vi "RDS Child Receive Message.vi"(8 "error in (no error)":errorcluster, 10 "RDS Message":refnum<class "RDS Message.lvclass">, 11 "RDS Test Child in":refnum<class "RDS Test Child.lvclass">) -> (0 "error out":errorcluster, 3 "RDS Test Child out":refnum<class "RDS Test Child.lvclass">)   [LabVIEW 2015, in "RDS Test Child.lvlib" / "RDS Test Child.lvclass"]
uses:
  RDS Test Child.lvclass
  Libraries/RDS Framework/RDS Message Class/RDS Message.lvclass
  Libraries/RDS Framework/RDS Message Class/RDS Message.lvclass/RDS Message.ctl
  Libraries/RDS Child Messages/AIP Status Message/AIP Status Response.lvclass
  Libraries/RDS Child Messages/AIP Status Message/AIP Status Response.lvclass/AIP Status Response.ctl
  RDS Test Child.lvclass/RDS Test Child.ctl
  Libraries/RDS Child Messages/GPS Data Message/GPS Data Message.lvclass
  Libraries/RDS Child Messages/GPS Data Message/GPS Data Message.lvclass/GPS Data Message.ctl
  Libraries/RDS Child Messages/State Sample Message/State Sample Message.lvclass
  Libraries/RDS Child Messages/State Sample Message/State Sample Message.lvclass/State Sample Message.ctl
  Libraries/RDS Child Messages/Helm/Helm Status Message/Helm Status Message.lvclass
  Libraries/RDS Child Messages/Helm/Helm Status Message/Helm Status Message.lvclass/Helm Status Message.ctl
  Libraries/RDS Child Messages/Depth Data Message/Depth Data Message.lvclass
  Libraries/RDS Child Messages/Depth Data Message/Depth Data Message.lvclass/Depth Data Message.ctl
  Libraries/RDS Child Messages/Battery Data/Battery Message.lvclass
  Libraries/RDS Child Messages/Battery Data/Battery Message.lvclass/Battery Message.ctl
  Libraries/RDS Child Messages/MCB/MCB Status Message/MCB Status.lvclass
  Libraries/RDS Child Messages/MCB/MCB Status Message/MCB Status.lvclass/MCB Status.ctl
  Libraries/RDS Child Messages/Compass/Compass Data Message.lvclass
  <vilib>/Utility/miscctls.llb/LV3DPointTypeDef.ctl
  Libraries/RDS Child Messages/Compass/Compass Data Message.lvclass/Compass Data Message.ctl
  Libraries/RDS Serial Handler/RDS Serial Frame.lvclass
  RDS State Tracker/RDS State/RDS State.lvclass
  Libraries/3rd Party/Artificial Horizon/lv-attitudecontrol.lvlib
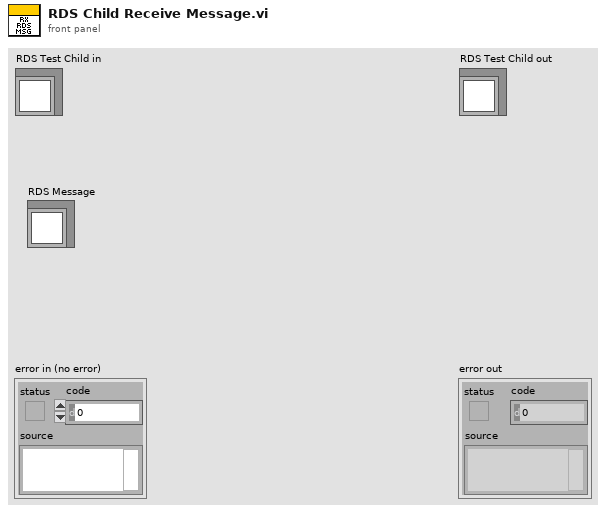
[diagram p1: front panel]
types:
  T1 = typedef "RDS Child Messages.lvlib/RDS Message ID.ctl" = enum16{"RDS Hello World", "String Message", "AIP_Status", "AIP_Command", "GPS_Data", "MCB_Command", "MCB_Status", "Compass_Data", "Depth_Data", "Battery_Data", "Contoller_State", "Set_Mag_Dev", "BTB_Shutdown", "State_Sample_Request", "State_Sample", "PID_Gains_Set", "Helm_Limiter_Set", "Helm_Heading_Command", "Helm_Steering_Command", "Helm_Status", "Controller_Message", "AIP_Set_Min_Depth", "Mission_Controller_State", "Mission_Upload", "Mission_Set_Op_and_Run", "Mission_Settings_Set"}
  T2 = typedef "LV3DPointTypeDef.ctl" = cluster{"X":sgl, "Y":sgl, "Z":sgl}
  T3 = typedef "RDS Instrument Library.lvlib/AIP Status.ctl" = cluster{"FWD Port":T4, "FWD Stbd":T4, "AFT Port":T4, "AFT Stbd":T4, "AIP Depth Min":u8}
  T4 = typedef "RDS Instrument Library.lvlib/AIP States.ctl" = enum16{"Deploy", "Deploying", "Deployed", "Stow", "Stowing", "Stowed", "Fault", "brakeOnStow", "breakOnDeploy", "Stopped", "Stopping"}
  T5 = typedef "RDS Libraries.lvlib/NMEA.lvlib/NMEA_GPRMC-data.ctl" = cluster{"TimeStamp":timestamp, "Validity":bool, "Latitude":dbl, "Latitude-Direction":T6, "Longitude":dbl, "Longitude-Direction":T7, "Speed in knots":sgl, "True course":sgl, "Date Stamp":timestamp, "Magnetic Variation (East/West)":sgl, "GPS Latitude":dbl, "GPS Longitude":dbl}
  T6 = typedef "RDS Libraries.lvlib/NMEA.lvlib/NMEA_LatitudeDirection.ctl" = enum16{"", "North", "South"}
  T7 = typedef "RDS Libraries.lvlib/NMEA.lvlib/NMEA_LongitudeDirection.ctl" = enum16{"", "East", "West"}
  T8 = typedef "RDS Child Messages.lvlib/Helm Status Control.ctl" = cluster{"Helm State":T9, "Heading Command Control":T10, "Steering Command Control":T11, "Last Command Time":timestamp, "Gains":T12, "Current Heading":dbl, "Port Throttle":i16, "STBD Throttle":i16, "Limiter":dbl}
  T9 = typedef "RDS Helm Actor.lvlib/Helm State.ctl" = enum16{"Idle", "Executing Heading Command", "Executing Steering Command"}
  T10 = typedef "RDS Child Messages.lvlib/Heading Command Cntrl.ctl" = cluster{"Throttle":i16, "Heading":sgl, "Duration (s)":i16}
  T11 = typedef "RDS Child Messages.lvlib/Steering Command Cntrl.ctl" = cluster{"Throttle":i16, "Rudder":i8, "Duration (s)":u16}
  T12 = typedef "RDS Child Messages.lvlib/PID Gains Control.ctl" = cluster{"P (Kc)":sgl, "I (Ti)":sgl, "D (Td)":sgl}
  T13 = typedef "RDS Child Messages.lvlib/Depth Data.ctl" = cluster{"Depth":sgl, "Water Temp":i8}
  T14 = typedef "RDS Instrument Library.lvlib/Battery Data.ctl" = cluster{"Battery Status":T15, "Pack Voltage":sgl, "Pack Current":sgl, "Pack Capacity":sgl, "Max Cell Temp":sgl, "Min Cell Temp":sgl, "Max Cell Voltage":sgl, "Min Cell Voltage":sgl}
  T15 = typedef "RDS Instrument Library.lvlib/Battery Status.ctl" = enum16{"Pack Normal", "Alarm: Cell temp too high", "Alarm: Pack voltage too high", "Warn: Pack voltage too high ", "Alarm: Pack voltage too low", "Warn: Pack voltage low", "Alarm Pack current too high", "Warn: Pack current too high ", "Fault: Pack to chassis connection detected", "Fault: Pack to cell connection error", "Fautl: System error"}
  T16 = typedef "RDS Child Messages.lvlib/MCB Motor Status.ctl" = cluster{"Motor Power":i16, "Motor Command":i16, "Battery Volts":sgl, "Battery Amps":sgl, "Motor Amps":sgl, "MCU Temp":i16, "Heatsink Temp":i16, "Fault Flags":u16, "StatusFlags":u16}
  T17 = typedef "RDS Child Messages.lvlib/MCB Channel.ctl" = enum16{"PORT", "STBD"}
  T18 = typedef "Throttles.ctl" = cluster{"Port":dbl, "STBD":dbl}
  T19 = typedef "RDS Instrument Library.lvlib/Compass Data.ctl" = cluster{"Compass Heading":sgl, "pitch Angle":sgl, "roll Angle":sgl, "Temperature":sgl, "Depth":sgl, "Magnetic Field":sgl, "Magnetic Field X":sgl, "Magnetic Field Y":sgl, "Magnetic Field Z":sgl, "Acceleration":sgl, "Acceleration X":sgl, "Acceleration Y":sgl, "Gyro":sgl, "Gyro X":sgl, "Acceleration Z":sgl, "Gyro Y":sgl, "Raw Heading":sgl}
  T20 = typedef "RDS Libraries.lvlib/lv-attitudecontrol.lvlib/AttitudeHandle.ctl" = cluster{"First Scene Object":refnum<vi>, "Drum":refnum<vi>, "Window":refnum<vi>, "Dial":refnum<vi>, "Scene Graph":refnum<vi>, "Last Drum Pitch":dbl, "Last Drum Roll ":dbl, "Last Dial Roll":dbl}
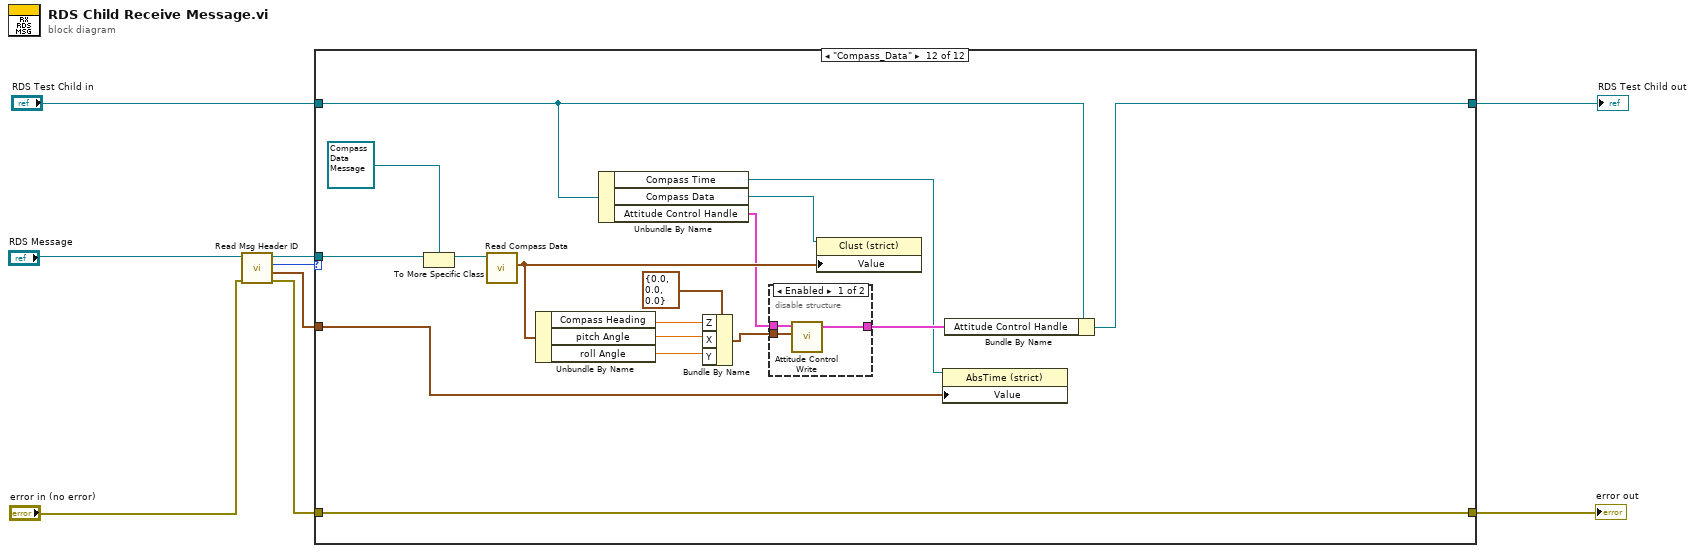
[diagram p0: block diagram]
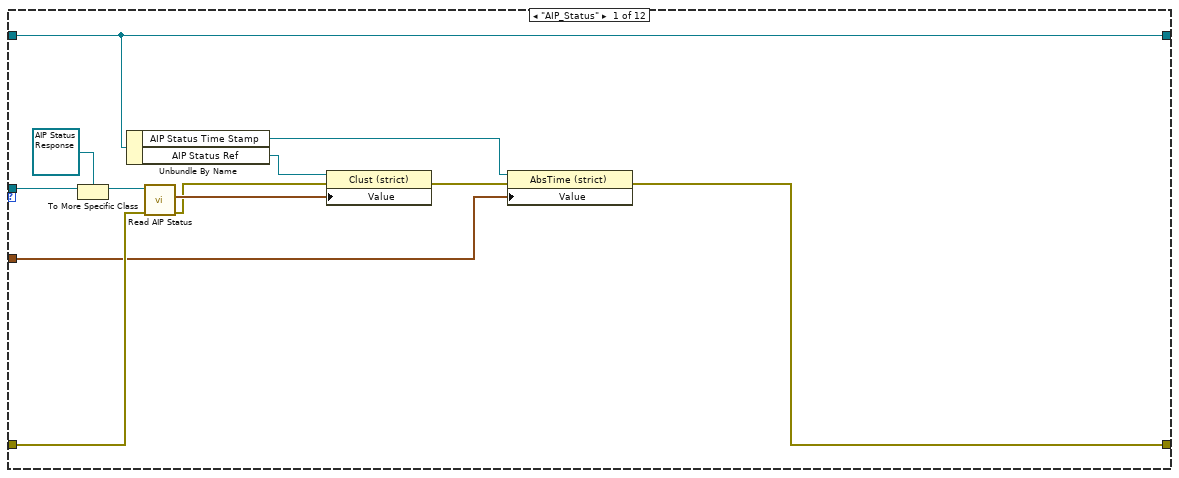
[diagram p2: hidden frame]
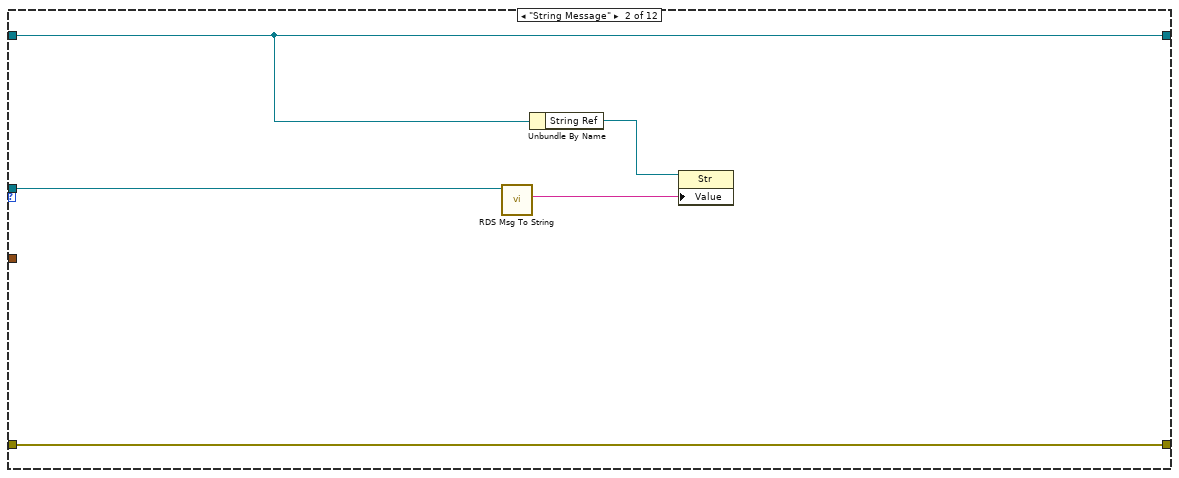
[diagram p3: hidden frame]
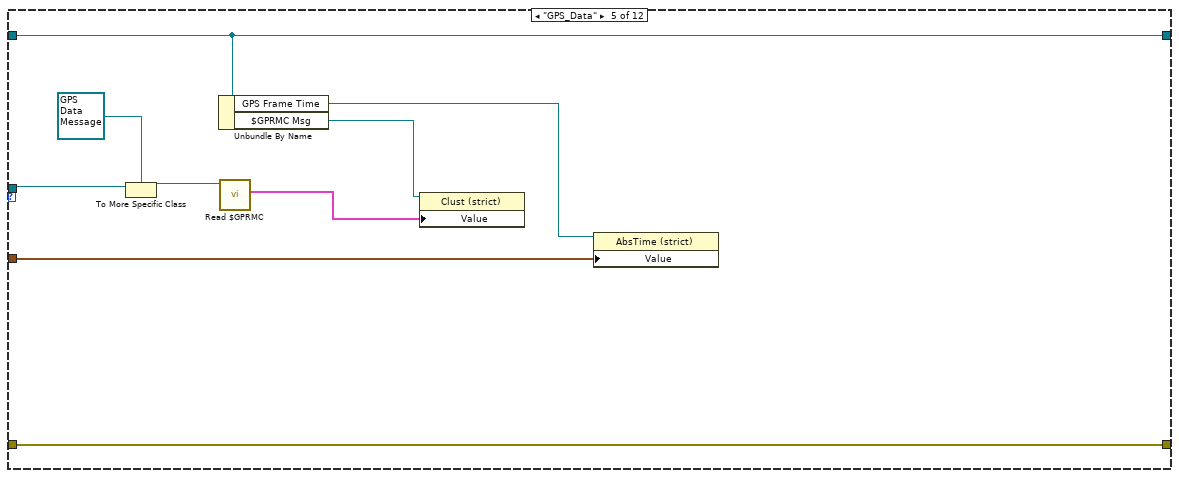
[diagram p6: hidden frame]
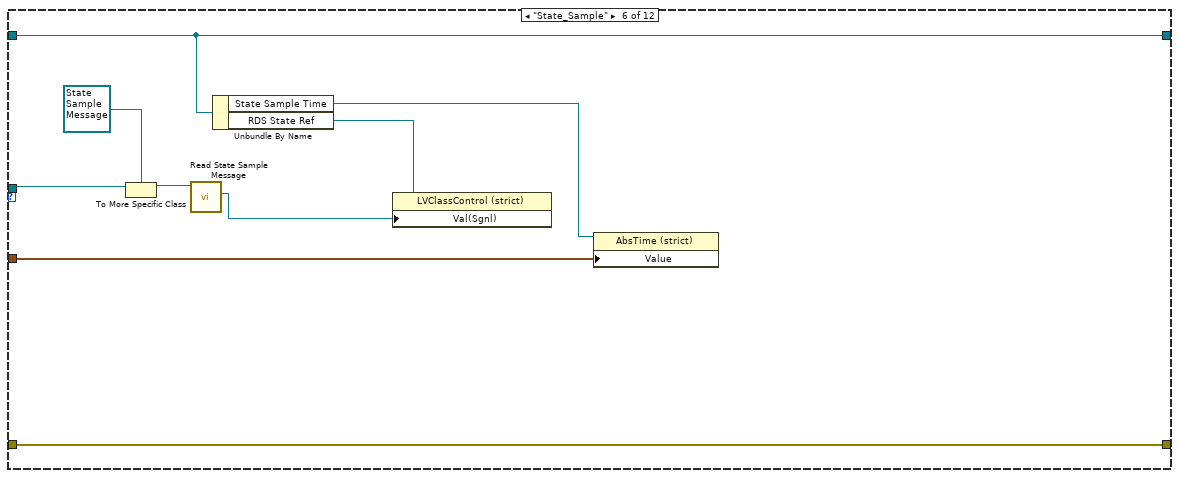
[diagram p7: hidden frame]
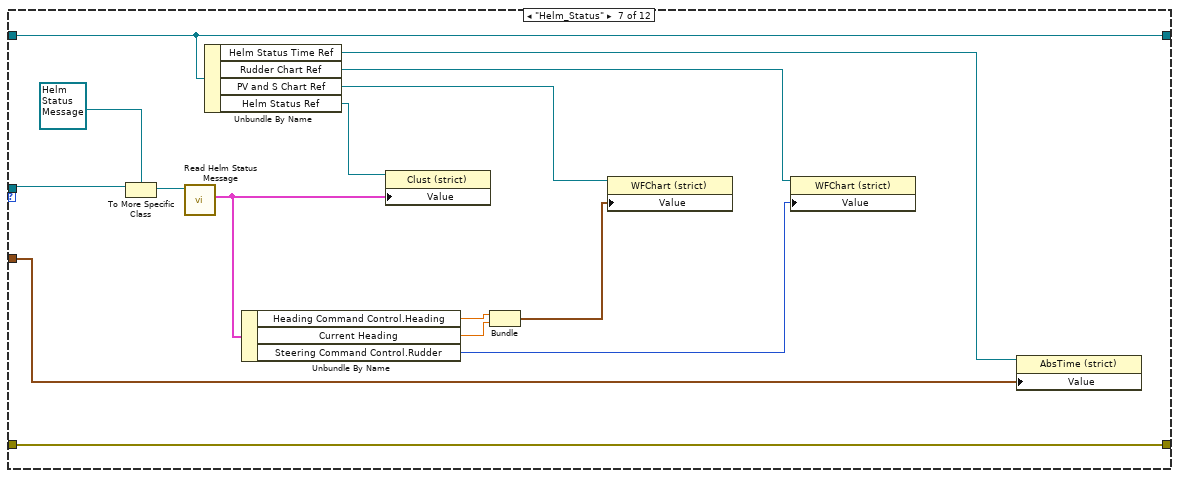
[diagram p8: hidden frame]
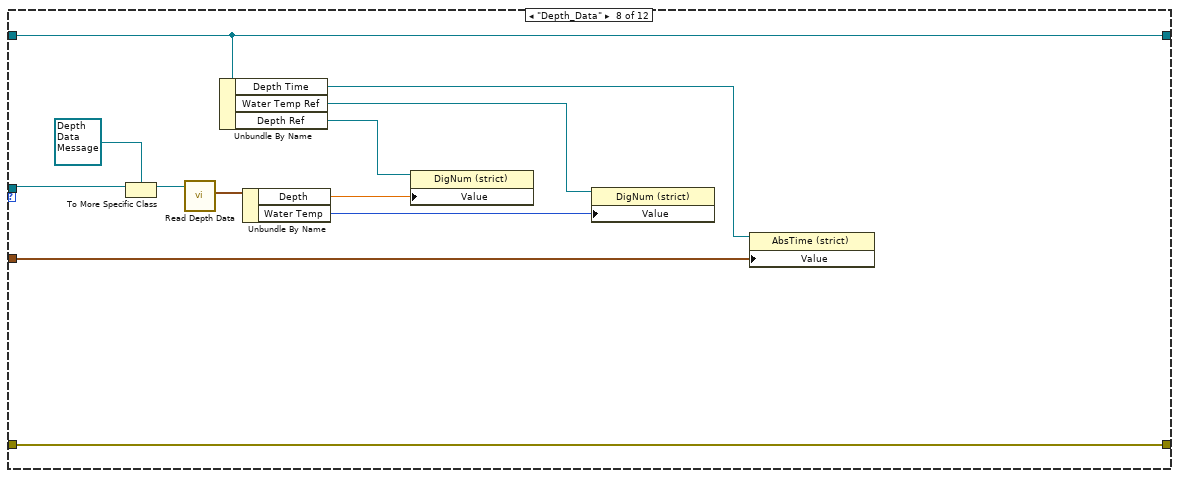
[diagram p9: hidden frame]
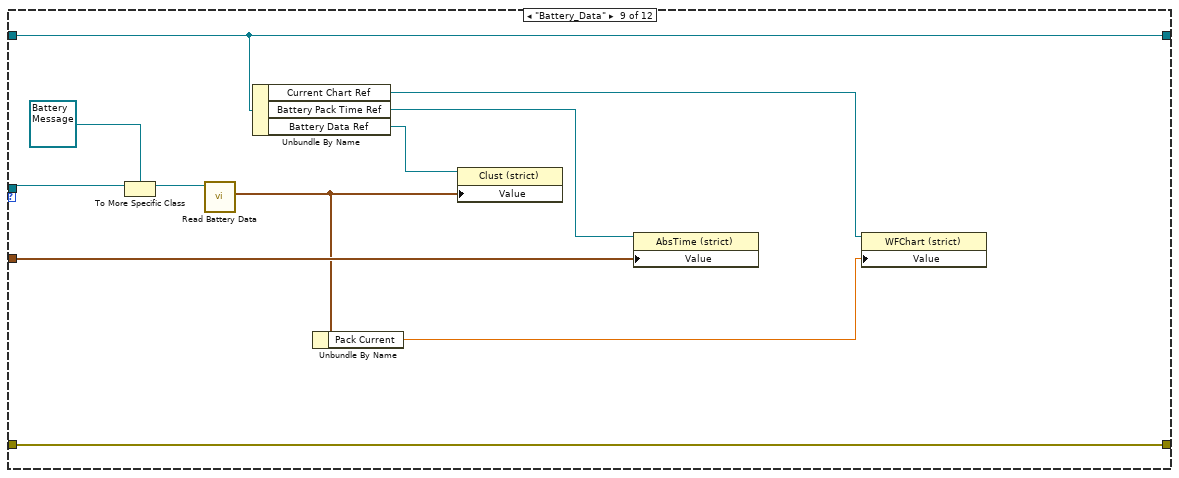
[diagram p10: hidden frame]
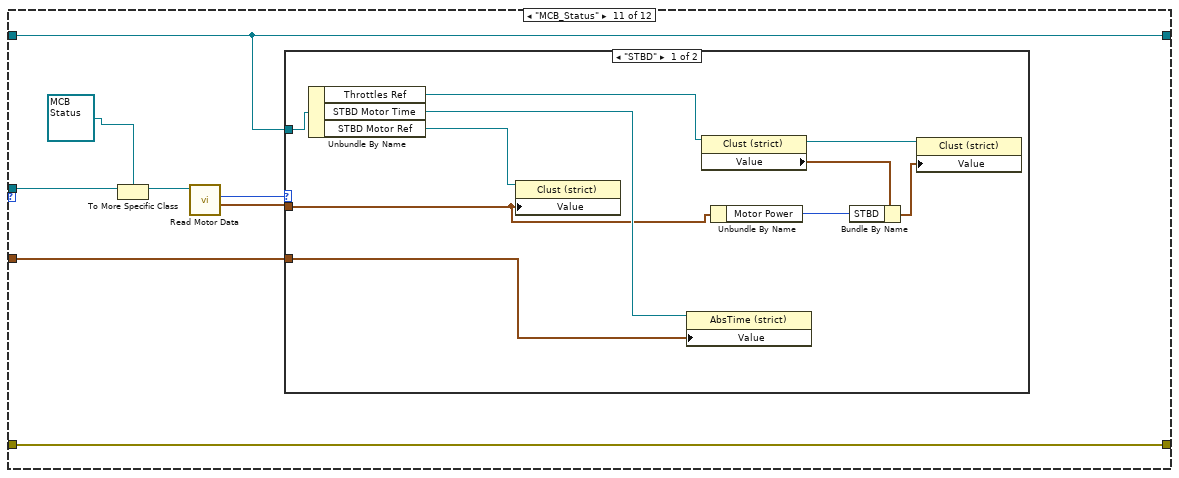
[diagram p12: hidden frame]
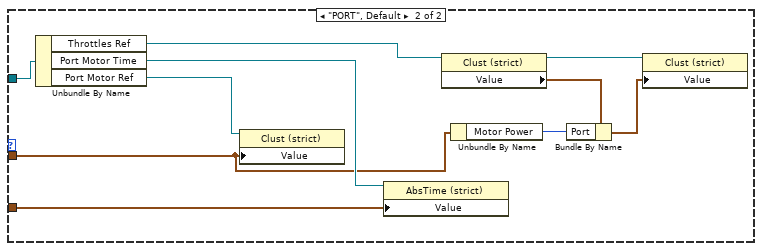
[diagram p13: hidden frame]
diagram:
  n1 = call "Read Msg Header ID.vi"("error in (no error)"="error in (no error)", "RDS Message in"="RDS Message") -> ("error out"=w3:errorcluster, "Time Stamp"=w4:timestamp, "Msg ID"=w7:T1, "RDS Message out"=w6:refnum<class "RDS Message.lvclass">)  [unwired: 5 in, 1 out]
  n2 = case shown="\"Compass_Data\"" w7 {
    tunnel: "RDS Test Child in" -> [w20 w23 w28 w30 w35 w46 w61 w73 w85 w88 w92 w120]
    tunnel: w6 -> [w17 w24 _ _ w38 w47 w62 w74 w82 _ w95 w132]
    tunnel: [w20 w23 w28 w30 w35 w46 w61 w73 w85 w88 w92 w119] -> w5
    tunnel: w4 -> [w13 _ _ _ w31 w43 w59 w64 w79 _ w89 w117]
    tunnel: w3 -> [w14 w22 w27 w29 w39 w48 w63 w75 w86 w87 w96 w133]
    tunnel: [w10 w22 w27 w29 w39 w48 w63 w75 w86 w87 w96 w133] -> w1
    frame "AIP_Status" {
      n3 = To More Specific Class(target class=refnum<class "AIP Status Response.lvclass"> refnum ("RDS Child Messages.lvlib:AIP Status Response.lvclass"), reference=w17) -> (specific class reference=w16:refnum<class "AIP Status Response.lvclass">)  [unwired: 1 in, 1 out]
      n4 = Unbundle By Name(w20) -> ("AIP Status Time Stamp"=w15:refnum<vi>, "AIP Status Ref"=w21:refnum<vi>)
      n5 = call "Read AIP Status.vi"("error in (no error)"=w14, "AIP Status Response in"=w16) -> ("error out"=w12:errorcluster, "AIP Status"=w19:T3)  [unwired: 6 in, 2 out]
      n6 = property class="Clust (strict)"(reference=w21, error in=w12, "Value"=w19) -> (error out=w11:errorcluster)  [unwired: 1 out]
      n7 = property class="AbsTime (strict)"(reference=w15, error in=w11, "Value"=w13) -> (error out=w10:errorcluster)  [unwired: 1 out]
    }
    frame "String Message" {
      n8 = call-dynamic "RDS Msg To String.vi"("RDS Message in"=w24) -> ("String"=w26:string)  [unwired: 8 in, 2 out]
      n9 = Unbundle By Name(w23) -> ("String Ref"=w25:refnum<vi>)
      n10 = property class="Str"(reference=w25, "Value"=w26) -> ()  [unwired: 1 in, 2 out]
    }
    frame "RDS Hello World", Default {
    }
    frame "AIP_Command" {
    }
    frame "GPS_Data" {
      n11 = To More Specific Class(target class=refnum<class "GPS Data Message.lvclass"> refnum ("RDS Child Messages.lvlib:GPS Data Message.lvclass"), reference=w38) -> (specific class reference=w36:refnum<class "GPS Data Message.lvclass">)  [unwired: 1 in, 1 out]
      n12 = Unbundle By Name(w35) -> ("GPS Frame Time"=w32:refnum<vi>, "$GPRMC Msg"=w34:refnum<vi>)
      n13 = call "Read $GPRMC.vi"("GPS Data Message in"=w36) -> ("GPRMC-data"=w33:T5)  [unwired: 8 in, 2 out]
      n14 = property class="Clust (strict)"(reference=w34, "Value"=w33) -> ()  [unwired: 1 in, 2 out]
      n15 = property class="AbsTime (strict)"(reference=w32, "Value"=w31) -> ()  [unwired: 1 in, 2 out]
    }
    frame "State_Sample" {
      n16 = To More Specific Class(target class=refnum<class "State Sample Message.lvclass"> refnum ("RDS Child Messages.lvlib:State Sample Message.lvclass"), reference=w47) -> (specific class reference=w41:refnum<class "State Sample Message.lvclass">)  [unwired: 1 in, 1 out]
      n17 = call "Read State Sample Message.vi"("State Sample Message in"=w41) -> ("State Sample"=w40:refnum<class "RDS State.lvclass">)  [unwired: 8 in, 2 out]
      n18 = Unbundle By Name(w46) -> ("State Sample Time"=w44:refnum<vi>, "RDS State Ref"=w45:refnum<vi>)
      n19 = property class="LVClassControl (strict)"(reference=w45, "Val(Sgnl)"=w40) -> ()  [unwired: 1 in, 2 out]
      n20 = property class="AbsTime (strict)"(reference=w44, "Value"=w43) -> ()  [unwired: 1 in, 2 out]
    }
    frame "Helm_Status" {
      n21 = To More Specific Class(target class=refnum<class "Helm Status Message.lvclass"> refnum ("RDS Child Messages.lvlib:Helm Status Message.lvclass"), reference=w62) -> (specific class reference=w57:refnum<class "Helm Status Message.lvclass">)  [unwired: 1 in, 1 out]
      n22 = call "Read Helm Status Message.vi"("Helm Status Message in"=w57) -> ("Helm Status"=w55:T8)  [unwired: 8 in, 2 out]
      n23 = Unbundle By Name(w61) -> ("Helm Status Time Ref"=w56:refnum<vi>, "Rudder Chart Ref"=w54:refnum<vi>, "PV and S Chart Ref"=w52:refnum<vi>, "Helm Status Ref"=w60:refnum<vi>)
      n24 = Unbundle By Name(w55) -> ("Heading Command Control.Heading"=w51:sgl, "Current Heading"=w50:dbl, "Steering Command Control.Rudder"=w53:i8)
      n25 = property class="Clust (strict)"(reference=w60, "Value"=w55) -> ()  [unwired: 1 in, 2 out]
      n26 = Bundle("Heading"=w51, "Current Heading"=w50) -> (w49:cluster{"Heading":sgl, "Current Heading":dbl})  [unwired: 1 in]
      n27 = property class="WFChart (strict)"(reference=w52, "Value"=w49) -> ()  [unwired: 1 in, 2 out]
      n28 = property class="WFChart (strict)"(reference=w54, "Value"=w53) -> ()  [unwired: 1 in, 2 out]
      n29 = property class="AbsTime (strict)"(reference=w56, "Value"=w59) -> ()  [unwired: 1 in, 2 out]
    }
    frame "Depth_Data" {
      n30 = To More Specific Class(target class=refnum<class "Depth Data Message.lvclass"> refnum ("RDS Child Messages.lvlib:Depth Data Message.lvclass"), reference=w74) -> (specific class reference=w70:refnum<class "Depth Data Message.lvclass">)  [unwired: 1 in, 1 out]
      n31 = call "Read Depth Data.vi"("Depth Data Message in"=w70) -> ("Depth Data"=w68:T13)  [unwired: 8 in, 2 out]
      n32 = Unbundle By Name(w73) -> ("Depth Time"=w65:refnum<vi>, "Water Temp Ref"=w69:refnum<vi>, "Depth Ref"=w72:refnum<vi>)
      n33 = Unbundle By Name(w68) -> ("Depth"=w67:sgl, "Water Temp"=w66:i8)
      n34 = property class="DigNum (strict)"(reference=w72, "Value"=w67) -> ()  [unwired: 1 in, 2 out]
      n35 = property class="DigNum (strict)"(reference=w69, "Value"=w66) -> ()  [unwired: 1 in, 2 out]
      n36 = property class="AbsTime (strict)"(reference=w65, "Value"=w64) -> ()  [unwired: 1 in, 2 out]
    }
    frame "Battery_Data" {
      n37 = To More Specific Class(target class=refnum<class "Battery Message.lvclass"> refnum ("RDS Child Messages.lvlib:Battery Message.lvclass"), reference=w82) -> (specific class reference=w81:refnum<class "Battery Message.lvclass">)  [unwired: 1 in, 1 out]
      n38 = call "Read Battery Data.vi"("Battery Message in"=w81) -> ("Battery Pack Info"=w77:T14)  [unwired: 8 in, 2 out]
      n39 = Unbundle By Name(w85) -> ("Current Chart Ref"=w78:refnum<vi>, "Battery Pack Time Ref"=w80:refnum<vi>, "Battery Data Ref"=w84:refnum<vi>)
      n40 = Unbundle By Name(w77) -> ("Pack Current"=w76:sgl)
      n41 = property class="Clust (strict)"(reference=w84, "Value"=w77) -> ()  [unwired: 1 in, 2 out]
      n42 = property class="AbsTime (strict)"(reference=w80, "Value"=w79) -> ()  [unwired: 1 in, 2 out]
      n43 = property class="WFChart (strict)"(reference=w78, "Value"=w76) -> ()  [unwired: 1 in, 2 out]
    }
    frame "MCB_Command" {
    }
    frame "MCB_Status" {
      n44 = To More Specific Class(target class=refnum<class "MCB Status.lvclass"> refnum ("RDS Child Messages.lvlib:MCB Status.lvclass"), reference=w95) -> (specific class reference=w93:refnum<class "MCB Status.lvclass">)  [unwired: 1 in, 1 out]
      n45 = call "Read Motor Data.vi"("MCB Status in"=w93) -> ("Motor Data"=w90:T16, "Motor"=w91:T17)  [unwired: 7 in, 2 out]
      n46 = case shown="\"STBD\"" w91 {
        tunnel: w92 -> [w105 w115]
        tunnel: w90 -> [w100 w109]
        tunnel: w89 -> [w104 w113]
        frame "STBD" {
          n47 = Unbundle By Name(w105) -> ("Throttles Ref"=w102:refnum<vi>, "STBD Motor Time"=w103:refnum<vi>, "STBD Motor Ref"=w106:refnum<vi>)
          n48 = property class="Clust (strict)"(reference=w106, "Value"=w100) -> ()  [unwired: 1 in, 2 out]
          n49 = property class="AbsTime (strict)"(reference=w103, "Value"=w104) -> ()  [unwired: 1 in, 2 out]
          n50 = property class="Clust (strict)"(reference=w102) -> (reference out=w97:refnum<vi>, "Value"=w101:T18)  [unwired: 1 in, 1 out]
          n51 = Unbundle By Name(w100) -> ("Motor Power"=w99:i16)
          n52 = Bundle By Name(cluster=w101, "STBD"=w99) -> (w98:T18)
          n53 = property class="Clust (strict)"(reference=w97, "Value"=w98) -> ()  [unwired: 1 in, 2 out]
        }
        frame "PORT", Default {
          n54 = Unbundle By Name(w115) -> ("Throttles Ref"=w110:refnum<vi>, "Port Motor Time"=w114:refnum<vi>, "Port Motor Ref"=w116:refnum<vi>)
          n55 = property class="Clust (strict)"(reference=w116, "Value"=w109) -> ()  [unwired: 1 in, 2 out]
          n56 = property class="AbsTime (strict)"(reference=w114, "Value"=w113) -> ()  [unwired: 1 in, 2 out]
          n57 = property class="Clust (strict)"(reference=w110) -> (reference out=w107:refnum<vi>, "Value"=w112:T18)  [unwired: 1 in, 1 out]
          n58 = Unbundle By Name(w109) -> ("Motor Power"=w111:i16)
          n59 = Bundle By Name(cluster=w112, "Port"=w111) -> (w108:T18)
          n60 = property class="Clust (strict)"(reference=w107, "Value"=w108) -> ()  [unwired: 1 in, 2 out]
        }
      }
    }
    frame "Compass_Data" {
      n61 = To More Specific Class(target class=refnum<class "Compass Data Message.lvclass"> refnum ("RDS Child Messages.lvlib:Compass Data Message.lvclass"), reference=w132) -> (specific class reference=w130:refnum<class "Compass Data Message.lvclass">)  [unwired: 1 in, 1 out]
      n62 = call "Read Compass Data.vi"("Compass Data Message in"=w130) -> ("Compass Data"=w128:T19)  [unwired: 8 in, 2 out]
      n63 = Unbundle By Name(w128) -> ("Compass Heading"=w125:sgl, "pitch Angle"=w124:sgl, "roll Angle"=w123:sgl)
      n64 = Unbundle By Name(w120) -> ("Compass Time"=w118:refnum<vi>, "Compass Data"=w129:refnum<vi>, "Attitude Control Handle"=w127:T20)
      n65 = Bundle By Name(cluster=T2 {"X"=0.0, "Y"=0.0, "Z"=0.0} ("pitch (x), roll (y), yaw (z)"), "Z"=w125, "X"=w124, "Y"=w123) -> (w122:T2)
      n66 = disable-structure shown="Enabled" {
        disable-tunnel: w127 -> [w136 w137]
        disable-tunnel: w122 -> [w135 _]
        disable-tunnel: [w134 w137] -> w121
        frame Enabled {
          n67 = call "Attitude Control Write.vi"("pitch (x), roll (y), yaw (z)"=w135, "Attitude Control Handle In"=w136) -> ("Attitude Control Handle Out"=w134:T20)  [unwired: 8 in, 1 out]
        }
        frame Disabled {
        }
      }
      n68 = property class="Clust (strict)"(reference=w129, "Value"=w128) -> ()  [unwired: 1 in, 2 out]
      n69 = property class="AbsTime (strict)"(reference=w118, "Value"=w117) -> ()  [unwired: 1 in, 2 out]
      n70 = Bundle By Name(cluster=w120, "Attitude Control Handle"=w121) -> (w119:refnum<class "RDS Test Child.lvclass">)
    }
  }
  "error out" <- w1
  "RDS Test Child out" <- w5
